vi "Save_Array_to_Spreadsheet.vi"() -> ()   [LabVIEW 2025]
uses:
  <vilib>/Utility/file.llb/Write Delimited Spreadsheet (DBL).vi
panel:
  in  "Stop":bool
  in  "Save":bool
  in  "Data":dbl[][](array[numeric])
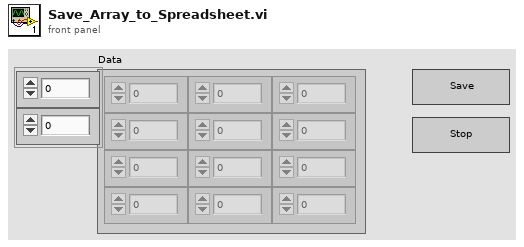
[diagram p1: front panel]
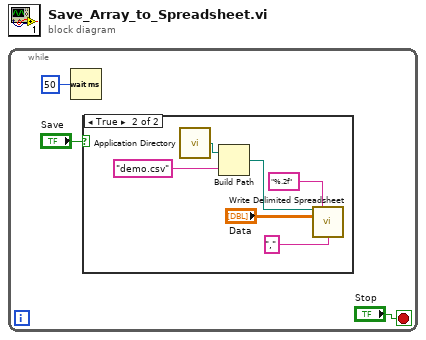
[diagram p0: block diagram]
diagram:
  n1 = while {
    stop <- "Stop" stop-if-true
    n2 = Wait (ms)(milliseconds to wait=u32 50) -> ()  [unwired: 1 out]
    n3 = case shown="True" "Save" {
      frame False {
      }
      frame True {
        n4 = call <vilib>:"Application Directory.vi"() -> ("Application Directory"=w8:path)
        n5 = Build Path(base path=w8, name or relative path="demo.csv") -> (appended path=w6:path)
        n6 = call-poly <vilib>:"Write Delimited Spreadsheet.vi"("file path (dialog if empty)"=w6, "format (%.3f)"="%.2f", "2D data"="Data", "delimiter (\\t)"="," ("delimiter (\\t)")) -> ()  [unwired: 10 in, 2 out]
      }
    }
  }
